vi "Get Async Processing Rates.vi"(8 "error in":errorcluster, 11 "custom device ref":T1 format="%.0x") -> (0 "error out":errorcluster, 1 "Outgoing Frame Rate":dbl caption="Outgoing frame processing rate [Hz]" min=0.0, 2 "Incoming Frame Rate":dbl caption="Incoming frame processing rate [Hz]" min=0.0, 3 "custom device ref out":T1 format="%.0x")   [LabVIEW 2020, in "AIM ARINC 664 Scripting.lvlib"]
uses:
  AIM ARINC 664 Scripting.lvlib
  <vilib>/NI VeriStand/Custom Device API/Custom Device Item Ref.ctl
  Constants.vi
  <vilib>/NI VeriStand/Custom Device API/Get Item Property (Double).vi
  <vilib>/NI VeriStand/Custom Device API/Custom Device API.lvlib
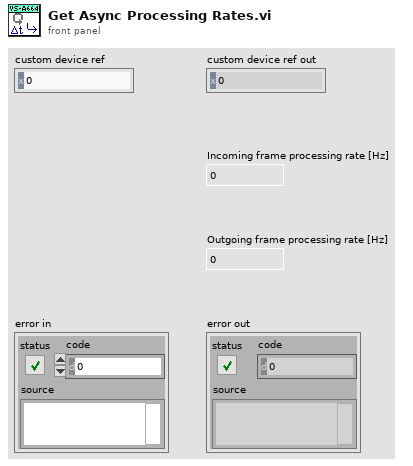
[diagram p1: front panel]
types:
  T1 = typedef "Custom Device API.lvlib/Custom Device Item Ref.ctl" = u64
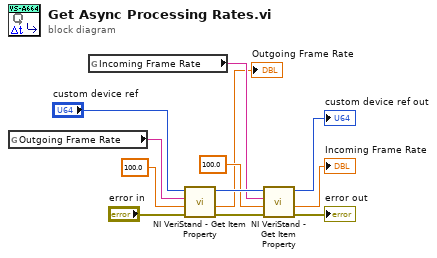
[diagram p0: block diagram]
diagram:
  n1 = global read "Constants.vi" "Outgoing Frame Rate"() -> (w6:string)
  n2 = global read "Constants.vi" "Incoming Frame Rate"() -> (w5:string)
  n3 = call-poly <vilib>:"NI VeriStand - Get Item Property.vi"("error in (no error)"="error in", "Default Value"=100.0, "Property Name"=w6, "Item Ref in"="custom device ref") -> ("error out"=w8:errorcluster, "Value"=→"Outgoing Frame Rate":dbl, "Item Ref out"=w11:T1)  [unwired: 4 in, 1 out]
  n4 = call-poly <vilib>:"NI VeriStand - Get Item Property.vi"("error in (no error)"=w8, "Default Value"=100.0, "Property Name"=w5, "Item Ref in"=w11) -> ("error out"=→"error out":errorcluster, "Value"=→"Incoming Frame Rate":dbl, "Item Ref out"=→"custom device ref out":T1)  [unwired: 4 in, 1 out]
